vi "eth-private-to-address.vi"(8 "error in (no error)":cluster{"状态":bool, "代码":i32, "源":string} caption="错误输入（无错误）", 11 "私钥输入":string="a9ddf02d9a749a49db0c29eef84fdbcf82e7f3e3c63d1c989c2118296439e9da") -> (0 "error out":cluster{"状态":bool, "代码":i32, "源":string} caption="错误输出", 1 "地址":string)   [LabVIEW 2020]
uses:
  C:/Program Files (x86)/National Instruments/LabVIEW 2020/examples/Connectivity/Python/support/PythonVersionsEnum.ctl
panel:
  in  "Python版本":T1=enum."3.6"
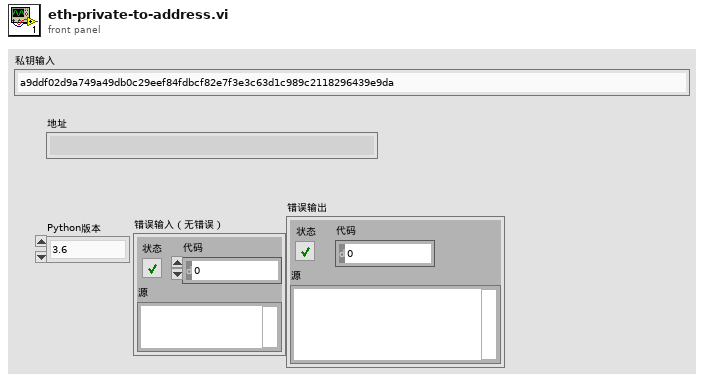
[diagram p1: front panel]
types:
  T1 = typedef "PythonVersionsEnum.ctl" = enum16{"2.7", "3.6"}
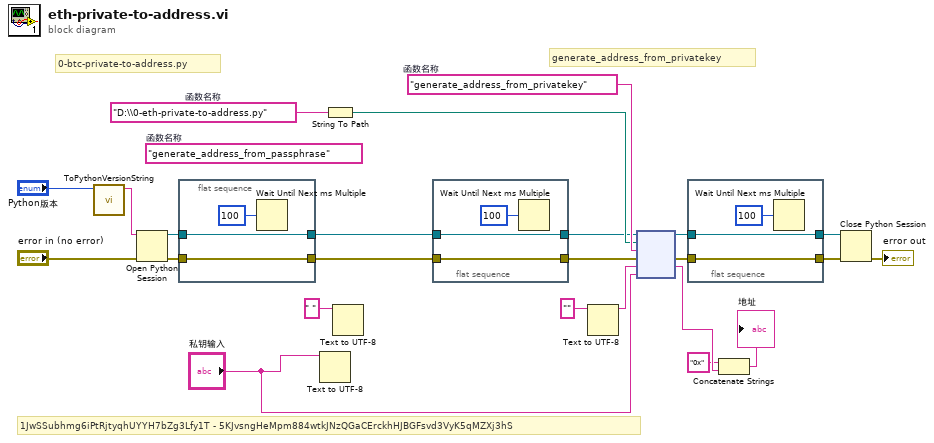
[diagram p0: block diagram]
diagram:
  w20 = "generate_address_from_privatekey"  # 函数名称
  (unwired) "generate_address_from_passphrase"  # 函数名称
  w21 = "D:\\0-eth-private-to-address.py"  # 函数名称
  # "generate_address_from_privatekey"
  # "0-btc-private-to-address.py"
  # "1JwSSubhmg6iPtRjtyqhUYYH7bZg3Lfy1T - 5KJvsngHeMpm884wtkJNzQGaCErckhHJBGFsvd3VyK5qMZXj3hS"
  n1 = call "ToPythonVersionString.vi"("Python版本"="Python版本") -> ("python版本字符串"=w24:string)  [unwired: 10 in]
  n2 = Open Python Session(python version=w24, 3:"error in (no error)") -> (session out=w18:refnum<k35>, error out=w10:errorcluster)  [unwired: 1 in]
  n3 = flat-sequence {
    tunnel: w18 -> [w26]
    tunnel: [w26] -> w4
    tunnel: [w25] -> w5
    tunnel: w10 -> [w25]
    frame #0 {
      n4 = Wait Until Next ms Multiple(millisecond multiple=u32 100 ("毫秒倍数")) -> ()  [unwired: 1 out]
    }
  }
  n5 = Text to UTF-8(11:"私钥输入") -> ()  [unwired: 2 in, 2 out]
  n6 = String To Path(string=w21) -> (path=w19:path)
  n7 = Text to UTF-8(11:" ") -> ()  [unwired: 2 in, 2 out]
  n8 = flat-sequence {
    tunnel: w4 -> [w29]
    tunnel: [w29] -> w17
    tunnel: [w28] -> w9
    tunnel: w5 -> [w28]
    frame #0 {
      n9 = Wait Until Next ms Multiple(millisecond multiple=u32 100 ("毫秒倍数")) -> ()  [unwired: 1 out]
    }
  }
  n10 = Text to UTF-8(11:"") -> (3:w11:string)  [unwired: 2 in, 1 out]
  n11 = node(w17, w19, w20, w9, w11, "私钥输入") -> (w14:refnum<k35>, w7:errorcluster, w3:string)  [unwired: 1 in, 2 out]
  n12 = flat-sequence {
    tunnel: [w32] -> w13
    tunnel: w14 -> [w32]
    tunnel: [w31] -> w8
    tunnel: w7 -> [w31]
    frame #0 {
      n13 = Wait Until Next ms Multiple(millisecond multiple=u32 100 ("毫秒倍数")) -> ()  [unwired: 1 out]
    }
  }
  n14 = Concatenate Strings("0x" ("字符串"), w3) -> (→"地址":string)
  n15 = Close Python Session(session in=w13, error in=w8) -> (11:→"error out":errorcluster)
